vi "INTELLIFAUCET DO Control.vi"(0 "VISA session":refnum<visa-resource-name>="MW100", 5 "HEWH MW100 Channel Numbers":T2="011", 7 "Normally Open":T1, 11 "Error In":errorcluster) -> (4 "dup VISA session":refnum<visa-resource-name>, 15 "error out":errorcluster)   [LabVIEW 2023]
uses:
  MW100/Type Definitions/HEWH MW100 Channel Numbers.ctl
  Type Definitions/HEWH Normally Open Valve Control.ctl
panel:
  # "PWR_MAIN: CLOSED = POWER OFF"
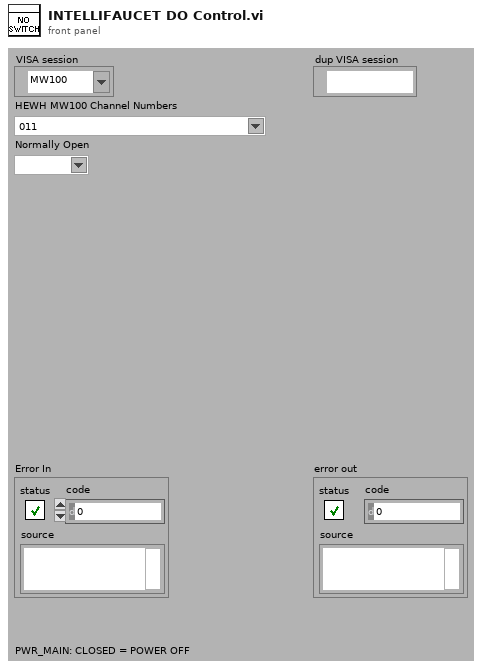
[diagram p1: front panel]
types:
  T1 = typedef "HEWH Normally Open Valve Control.ctl" = string
  T2 = typedef "HEWH MW100 Channel Numbers.ctl" = string
  T3 = enum8{"Affirmative", "Single Negative", "Multiple Negative", "ASCII", "BINARY", "END"}
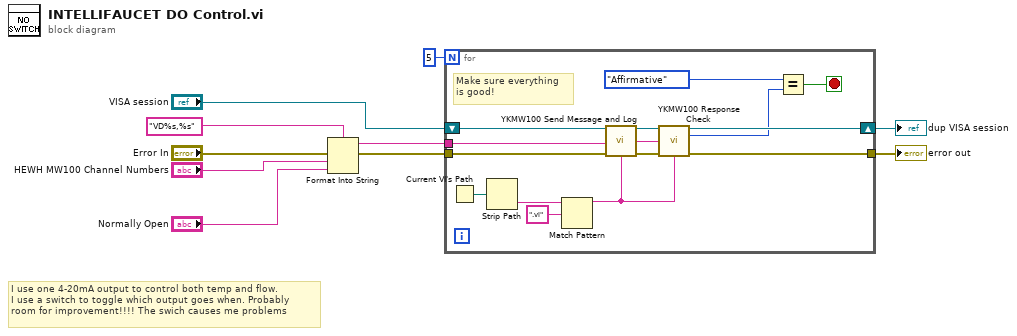
[diagram p0: block diagram]
diagram:
  # "I use one 4-20mA output to control both temp and flow.\nI use a switch to toggle which output goes when. Probably\nroom for improvement!!!! The swich causes me problems"
  n1 = Format Into String(format string="VD%s,%s", error in="Error In", "HEWH MW100 Channel Numbers", "Normally Open") -> (resulting string=w3:string, error out=w6:errorcluster)  [unwired: 1 in]
  n2 = for {
    N: 5 -> [_]
    tunnel: w3 -> [w18]
    shift-right: [w24] -> w9
    shift-left: "VISA session" -> [w25]
    tunnel: w6 -> [w22]
    tunnel: [w23] -> w8
    stop <- w17 stop-if-true
    # "Make sure everything \nis good!"
    n3 = Current VI's Path() -> (path=w13:path)
    n4 = Strip Path(path=w13) -> (name=w14:string)  [unwired: 1 out]
    n5 = Match Pattern(string=w14, regular expression=".vi") -> (before substring=w11:string)  [unwired: 1 in, 3 out]
    n6 = call "YKMW100 Send Message and Log.vi"("VISA session"=w25, "Send Message (\"\")"=w18, "error in (no error)"=w22, "Source (\"\")"=w11) -> ("dup VISA session"=w21:refnum<visa-resource-name>, "Read Buffer"=w19:string, "error out"=w20:errorcluster)  [unwired: 9 in]
    n7 = call "YKMW100 Response Check.vi"("VISA session"=w21, "Message In (\"\")"=w19, "error in (no error)"=w20, "Source (\"\")"=w11) -> ("dup VISA session"=w24:refnum<visa-resource-name>, "Response Type"=w16:T3, "error out"=w23:errorcluster)  [unwired: 7 in, 2 out]
    n8 = Equal?(x=T3."Affirmative", y=w16) -> (x = y?=w17:bool)
  }
  "dup VISA session" <- w9
  "error out" <- w8
